vi "Set Cell Data.vi"(4 "Ref. Value":string, 6 "Ref. Header":string, 8 "error in (no error)":errorcluster, 9 "Cell Data":string, 10 "Cell Header":string, 11 "SLL Spreadsheet in":refnum<class "SLL Table.lvclass">) -> (0 "error out":errorcluster, 3 "SLL Spreadsheet out":refnum<class "SLL Table.lvclass">)   [LabVIEW 2014, in "SLL Table.lvclass"]
uses:
  SLL Table.lvclass
  SLL Table.lvclass/SLL Table.ctl
panel:
  out "Header Present?":bool
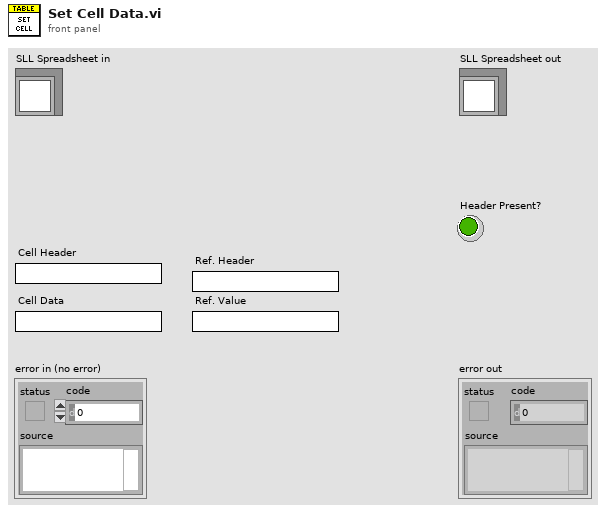
[diagram p1: front panel]
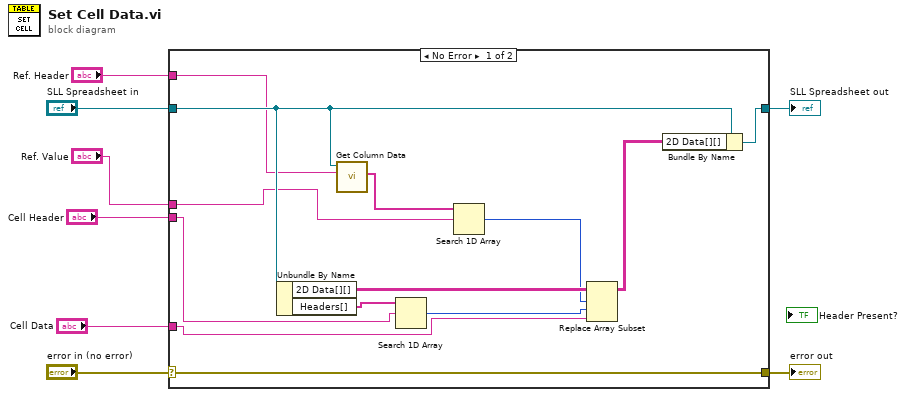
[diagram p0: block diagram]
diagram:
  n1 = case shown="No Error" "error in (no error)" {
    selector: "error in (no error)" -> [w21 w23]
    tunnel: [w21 w23] -> w7
    tunnel: [w12 w22] -> w5
    tunnel: "SLL Spreadsheet in" -> [w13 w22]
    tunnel: "Cell Header" -> [w18 _]
    tunnel: "Cell Data" -> [w14 _]
    tunnel: "Ref. Header" -> [w10 _]
    tunnel: "Ref. Value" -> [w9 _]
    frame No Error {
      n2 = Unbundle By Name(w13) -> ("2D Data[][]"=w17:string[][], "Headers[]"=w19:string[])
      n3 = call "Get Column Data.vi"("Header"=w10, "SLL Spreadsheet in"=w13) -> ("Data[]"=w20:string[])  [unwired: 6 in, 3 out]
      n4 = Search 1D Array(1D array=w19, element=w18) -> (index of element=w15:i32)  [unwired: 1 in]
      n5 = Search 1D Array(1D array=w20, element=w9) -> (index of element=w16:i32)  [unwired: 1 in]
      n6 = Replace Array Subset(array=w17, new element=w14, index (row)=w16, index (col)=w15) -> (w11:string[][])
      n7 = Bundle By Name(cluster=w13, "2D Data[][]"=w11) -> (w12:refnum<class "SLL Table.lvclass">)
    }
    frame Error {
    }
  }
  "error out" <- w7
  "SLL Spreadsheet out" <- w5
